vi "Unitary_Test_Stop.vi"() -> (0 "Test_passed":bool)   [LabVIEW 2015]
panel:
  out "hidden 2":errorcluster
  out "error 2 must FAIL":errorcluster={"status"=TRUE, "code"=0, "source"="\nClose error on expID:TestNO_STOP\nExperience aborted"}
  out "hidden2":errorcluster
  out "hidden3 2":errorcluster
  in  "Experience ID1 2":string="TestNO_STOP"
  out "error 1 must be OK":errorcluster
  out "error out":errorcluster
  out "hidden3":errorcluster
  out "hidden":errorcluster
  in  "Experience ID1":string="TestOK"
  out "Test_OK":bool[](array[boolean])
  # "Test basic methods with some testing plant"
  # "TestNO_STOP"
  # "This test take time because a vi refuses to close\n(its part of the test)"
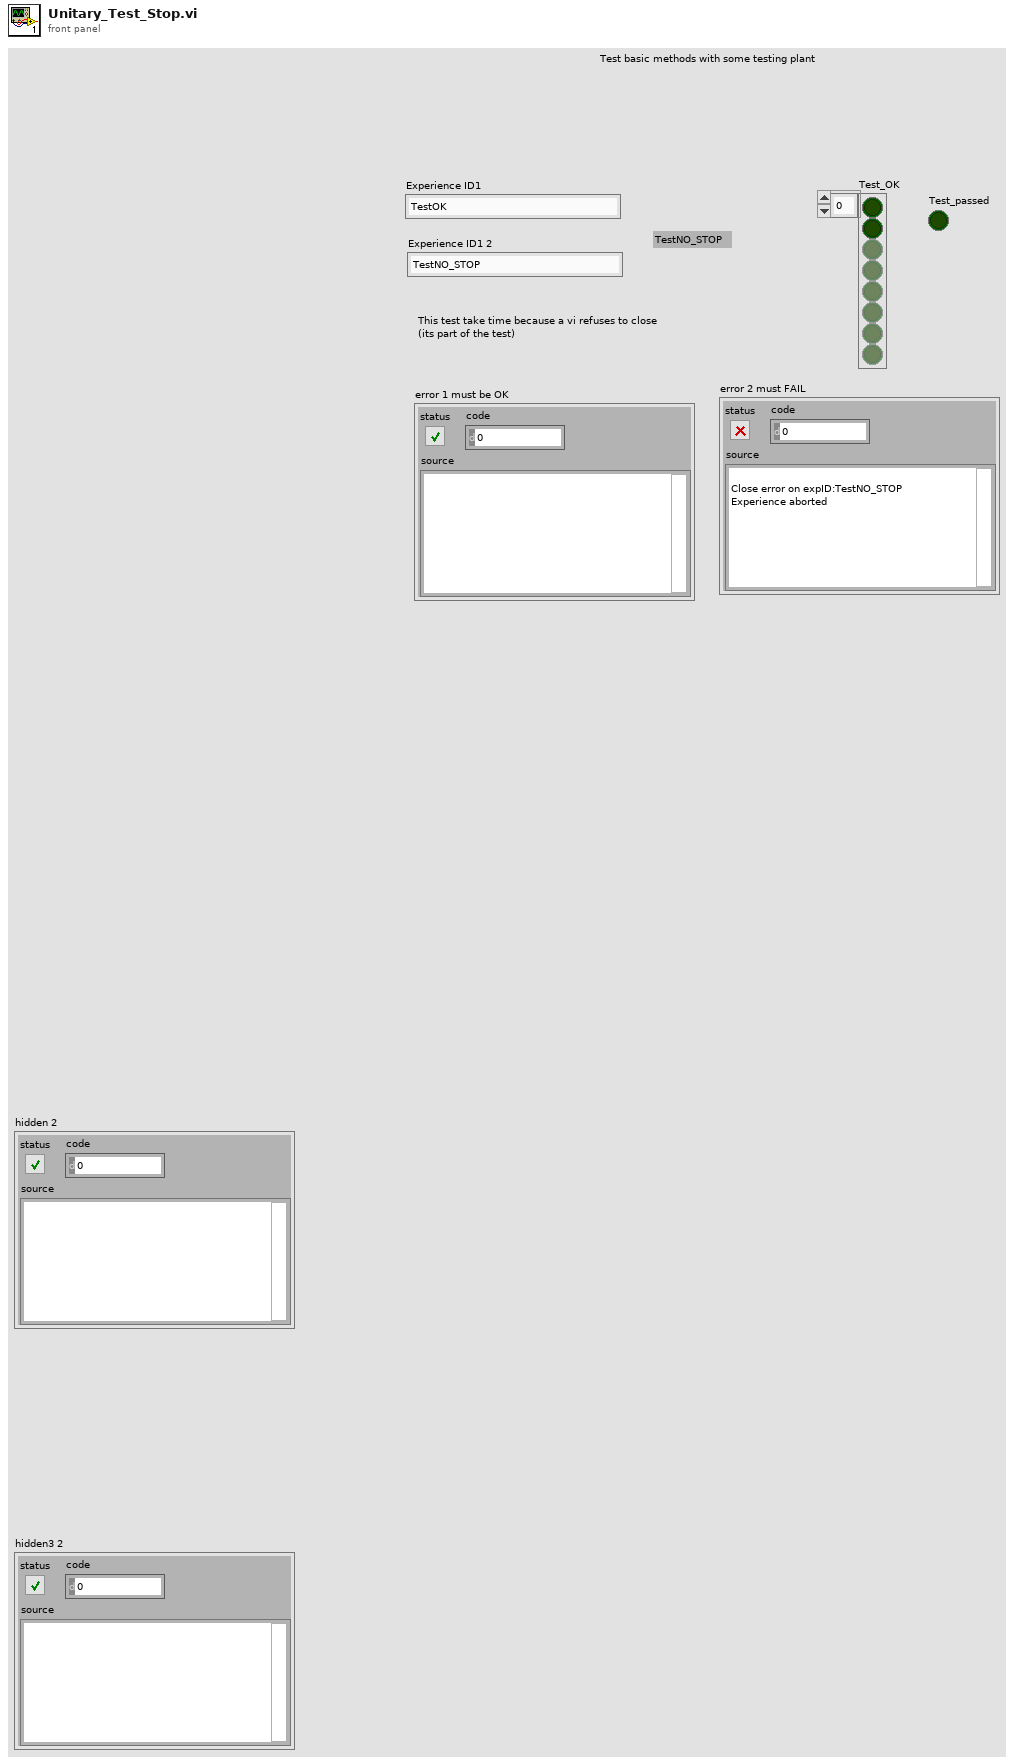
[diagram p1: front panel]
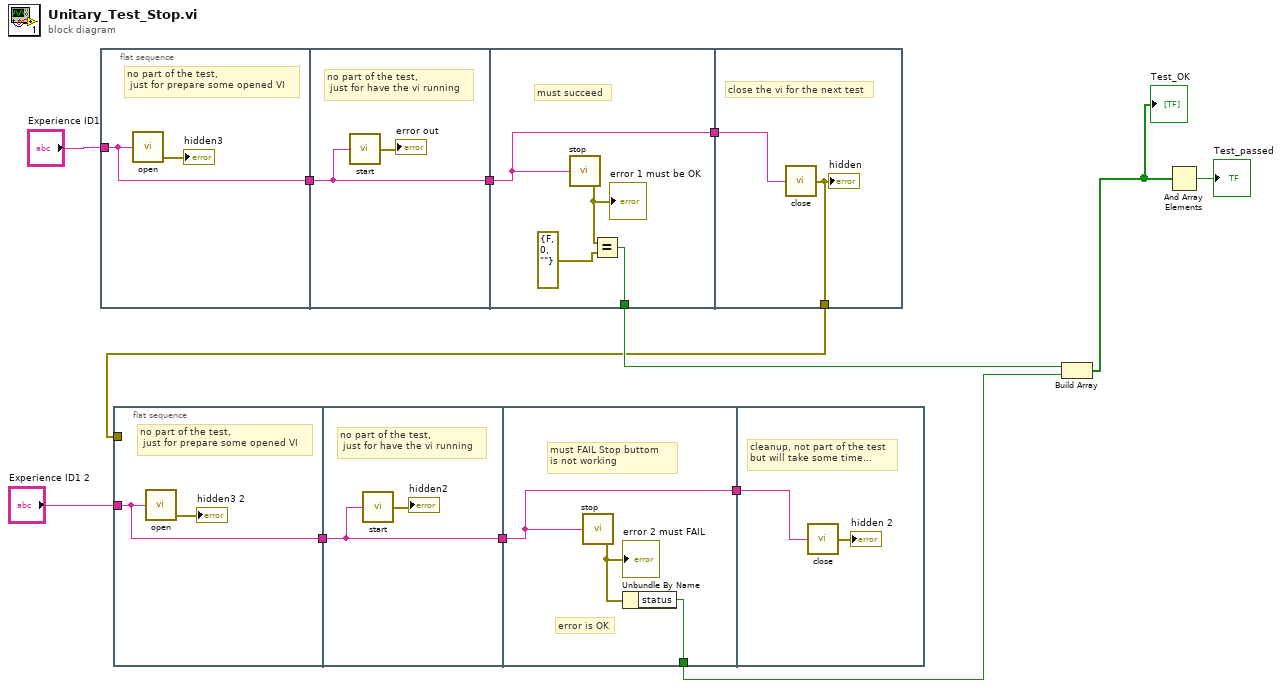
[diagram p0: block diagram]
diagram:
  n1 = flat-sequence {
    tunnel: "Experience ID1" -> [w15]
    tunnel: [w15] -> w9
    tunnel: w9 -> [w17]
    tunnel: [w17] -> w8
    tunnel: w8 -> [w19]
    tunnel: [w19] -> w10
    tunnel: [w20] -> w11
    tunnel: w10 -> [w23]
    tunnel: [w22] -> w1
    frame #0 {
      # "no part of the test,\n just for prepare some opened VI"
      n2 = call "open.vi"("Experience ID"=w15) -> ("error out"=→"hidden3":errorcluster)  [unwired: 2 out]
    }
    frame #1 {
      # "no part of the test,\n just for have the vi running"
      n3 = call "start.vi"("Experience ID"=w17) -> ("error out"=→"error out":errorcluster)
    }
    frame #2 {
      # "must succeed"
      n4 = call "stop.vi"("Experience ID"=w19) -> ("error out"=w18:errorcluster)
      "error 1 must be OK" <- w18
      n5 = Equal?(x=w18, y=errorcluster {"status"=FALSE, "code"=0, "source"=""} ("error out")) -> (x = y?=w20:bool)
    }
    frame #3 {
      # "close the vi for the next test"
      n6 = call "close.vi"("Experience ID"=w23) -> ("error out"=w22:errorcluster)
      "hidden" <- w22
    }
  }
  n7 = flat-sequence {
    tunnel: "Experience ID1 2" -> [w25]
    tunnel: [w25] -> w6
    tunnel: w1 -> [_]
    tunnel: w6 -> [w27]
    tunnel: [w27] -> w5
    tunnel: w5 -> [w30]
    tunnel: [w30] -> w4
    tunnel: [w28] -> w2
    tunnel: w4 -> [w31]
    frame #0 {
      # "no part of the test,\n just for prepare some opened VI"
      n8 = call "open.vi"("Experience ID"=w25) -> ("error out"=→"hidden3 2":errorcluster)  [unwired: 2 out]
    }
    frame #1 {
      # "no part of the test,\n just for have the vi running"
      n9 = call "start.vi"("Experience ID"=w27) -> ("error out"=→"hidden2":errorcluster)
    }
    frame #2 {
      # "error is OK"
      # "must FAIL Stop buttom \nis not working"
      n10 = call "stop.vi"("Experience ID"=w30) -> ("error out"=w29:errorcluster)
      "error 2 must FAIL" <- w29
      n11 = Unbundle By Name(w29) -> ("status"=w28:bool)
    }
    frame #3 {
      # "cleanup, not part of the test\nbut will take some time..."
      n12 = call "close.vi"("Experience ID"=w31) -> ("error out"=→"hidden 2":errorcluster)
    }
  }
  n13 = Build Array(w11, w2) -> (w7:bool[])
  "Test_OK" <- w7
  n14 = And Array Elements(Boolean array=w7) -> (logical AND=→"Test_passed":bool)
